vi "Trapu16toDbl.vi"(9 "Detector Type":string, 10 "Trap Sets":u32, 11 "Raw Trap Data In":i16[](array[numeric])) -> (0 "Channel pattern":i32, 1 "Channel Names":string[](array[string]), 2 "Trap Data":dbl[][](array[numeric]), 3 "Trap Data Out":i16[](array[numeric]))   [LabVIEW 2013]
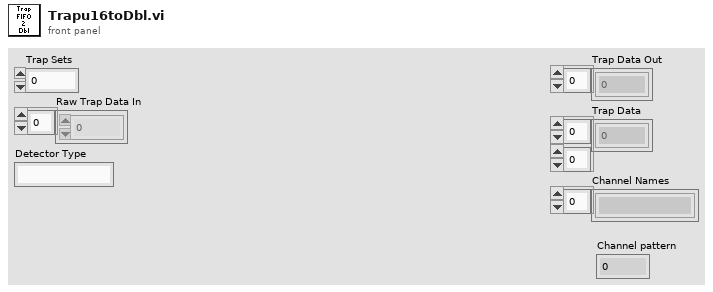
[diagram p1: front panel]
types:
  T1 = cluster{string, string, string, string, string, string, string, string}
  T2 = cluster{string, string, string, string, string, string, string, string, string, string, string, string}
  T3 = cluster{string, string, string, string, string, string, string, string, string, string, string, string, string}
  T4 = cluster{string, string, string, string, string, string, string, string, string, string, string, string, string, string}
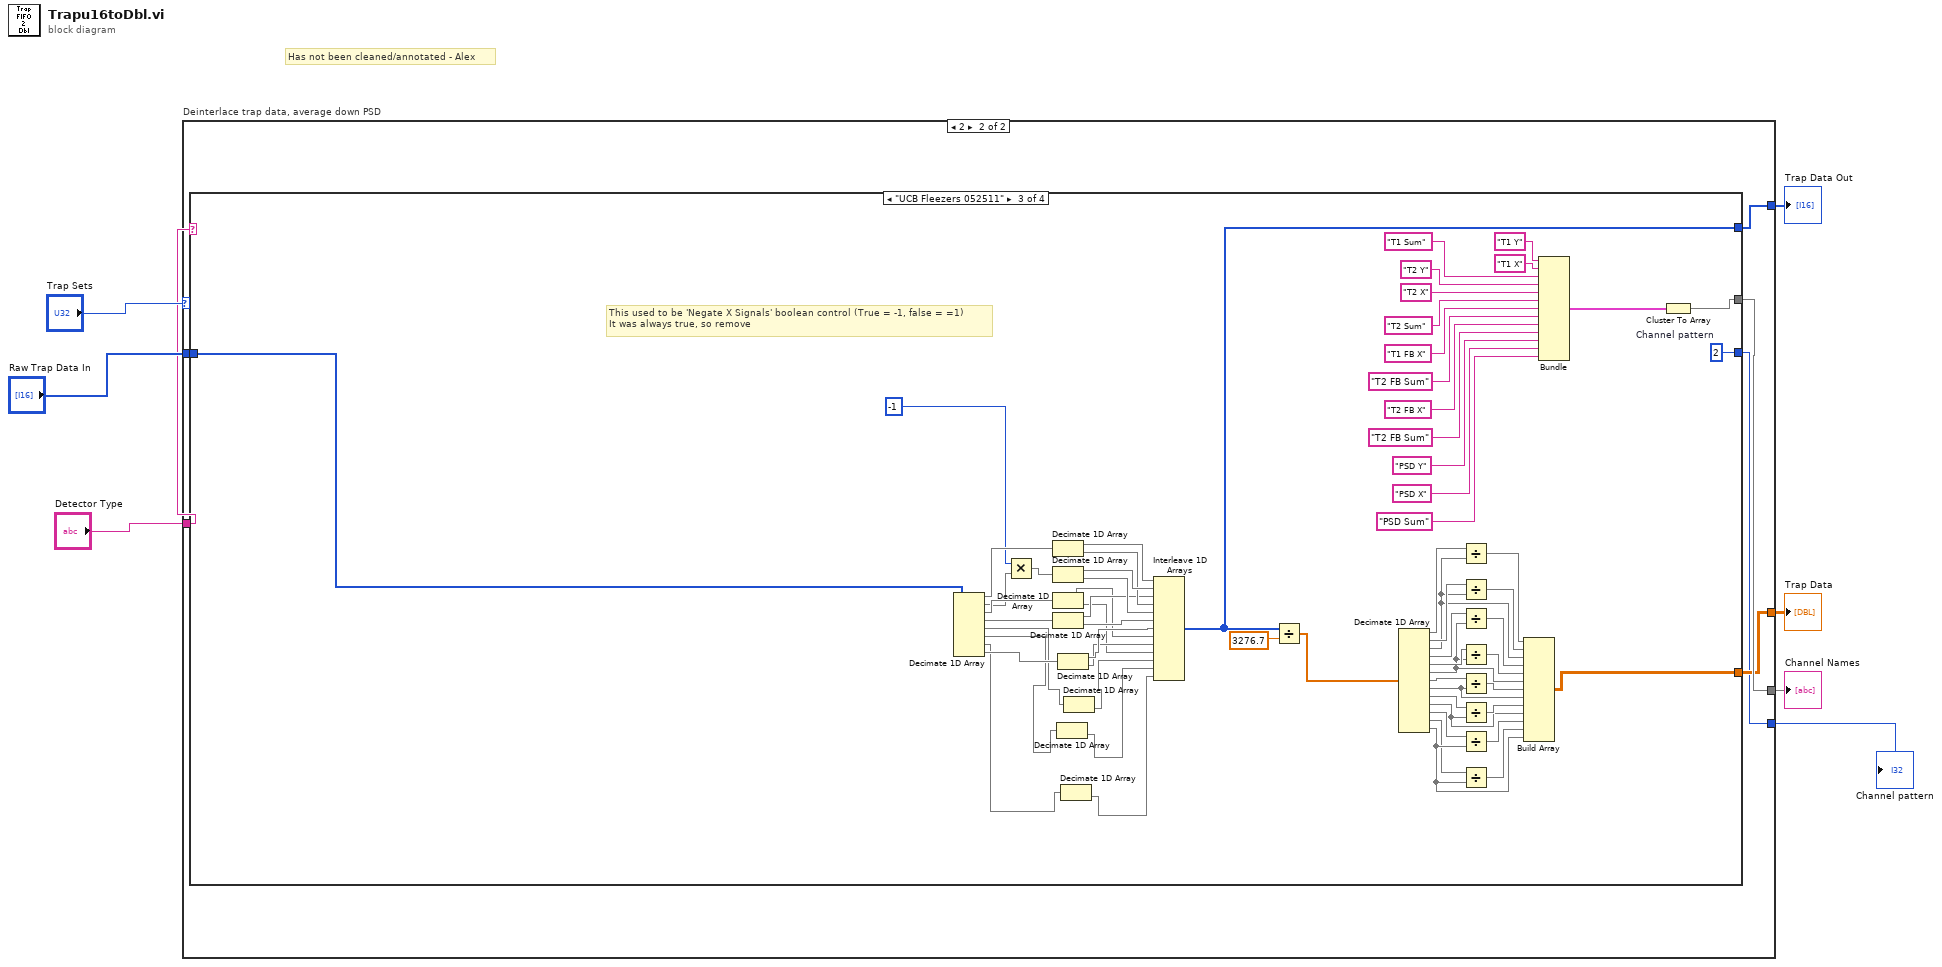
[diagram p0: block diagram]
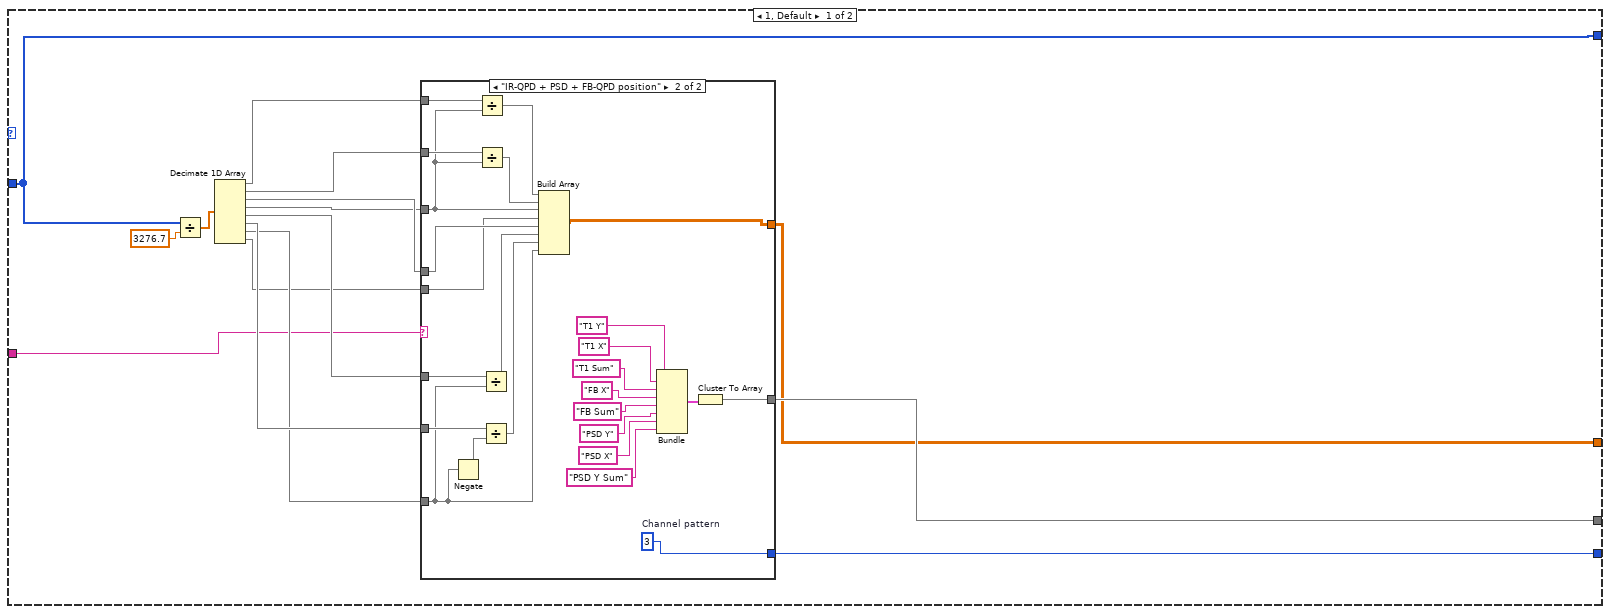
[diagram p2: hidden frame]
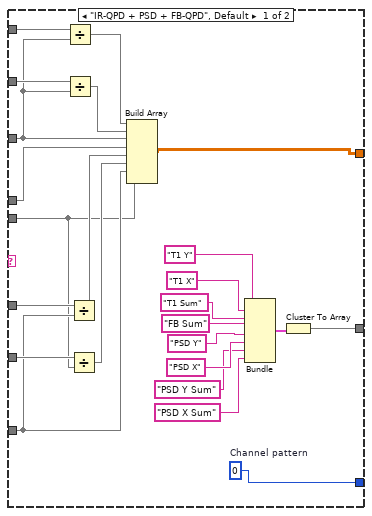
[diagram p3: hidden frame]
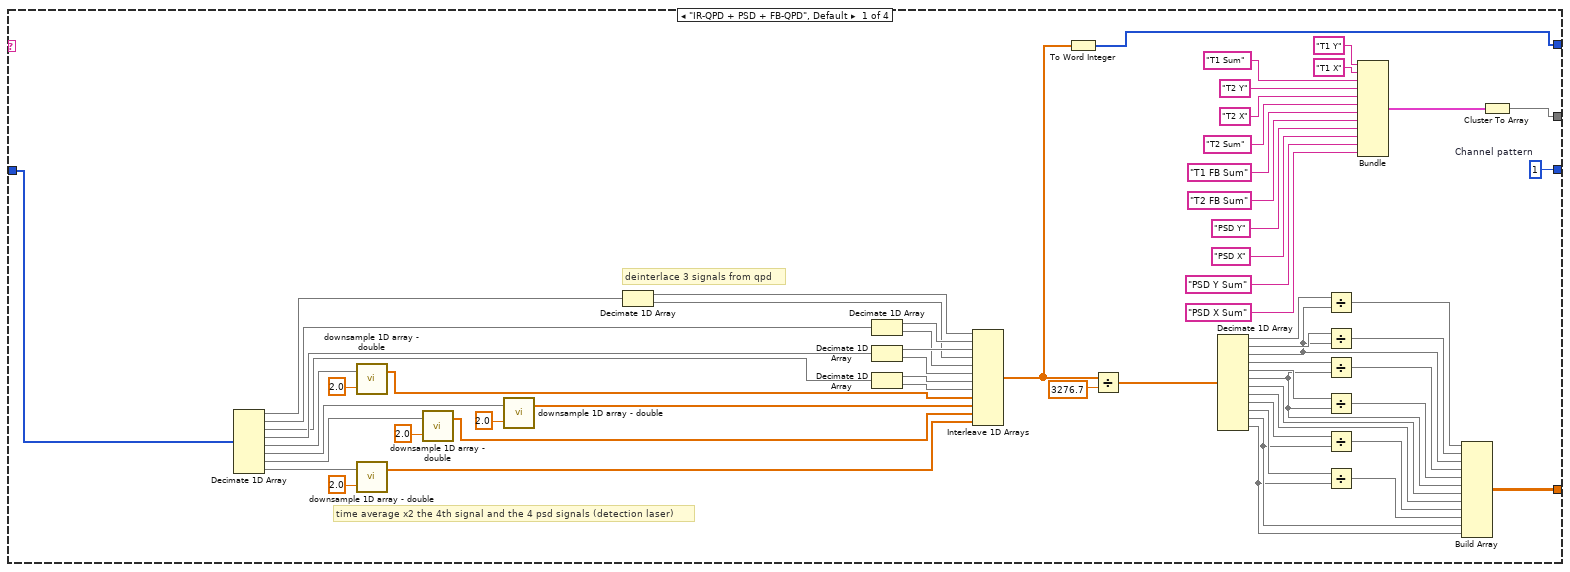
[diagram p4: hidden frame]
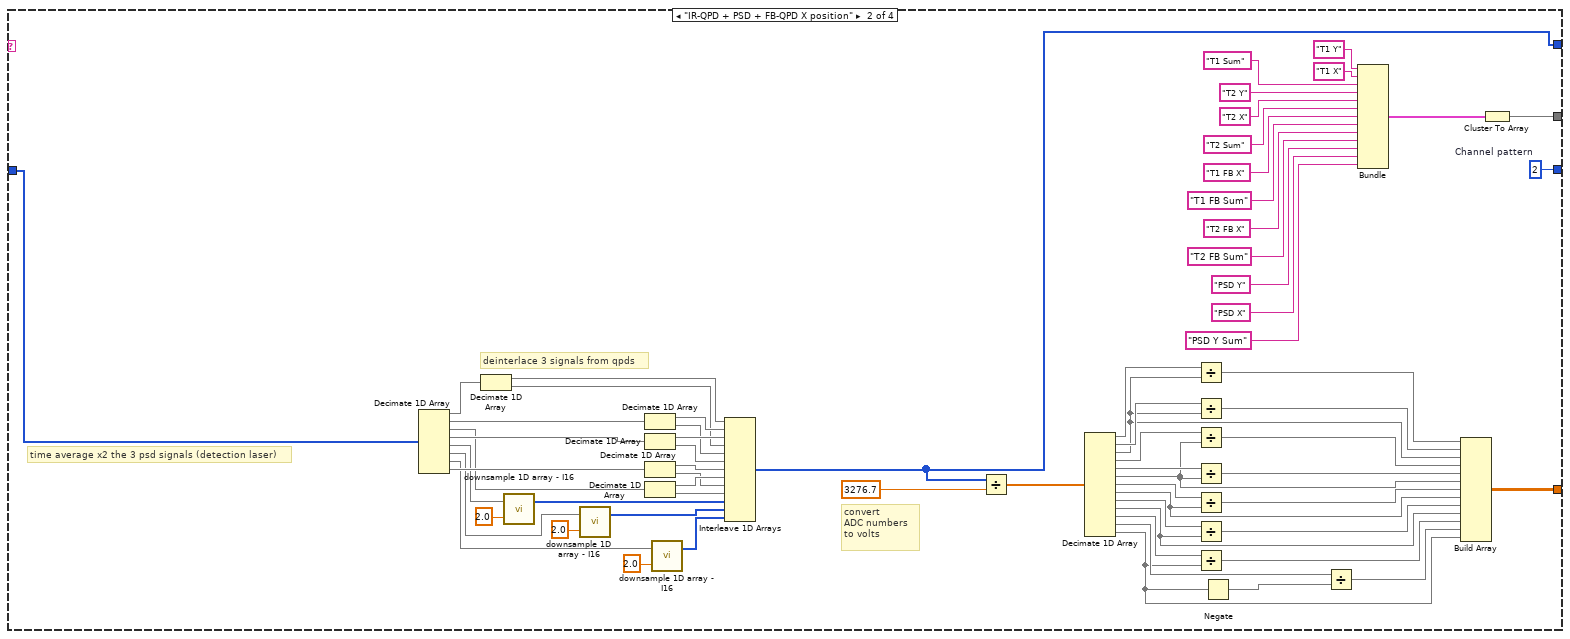
[diagram p5: hidden frame]
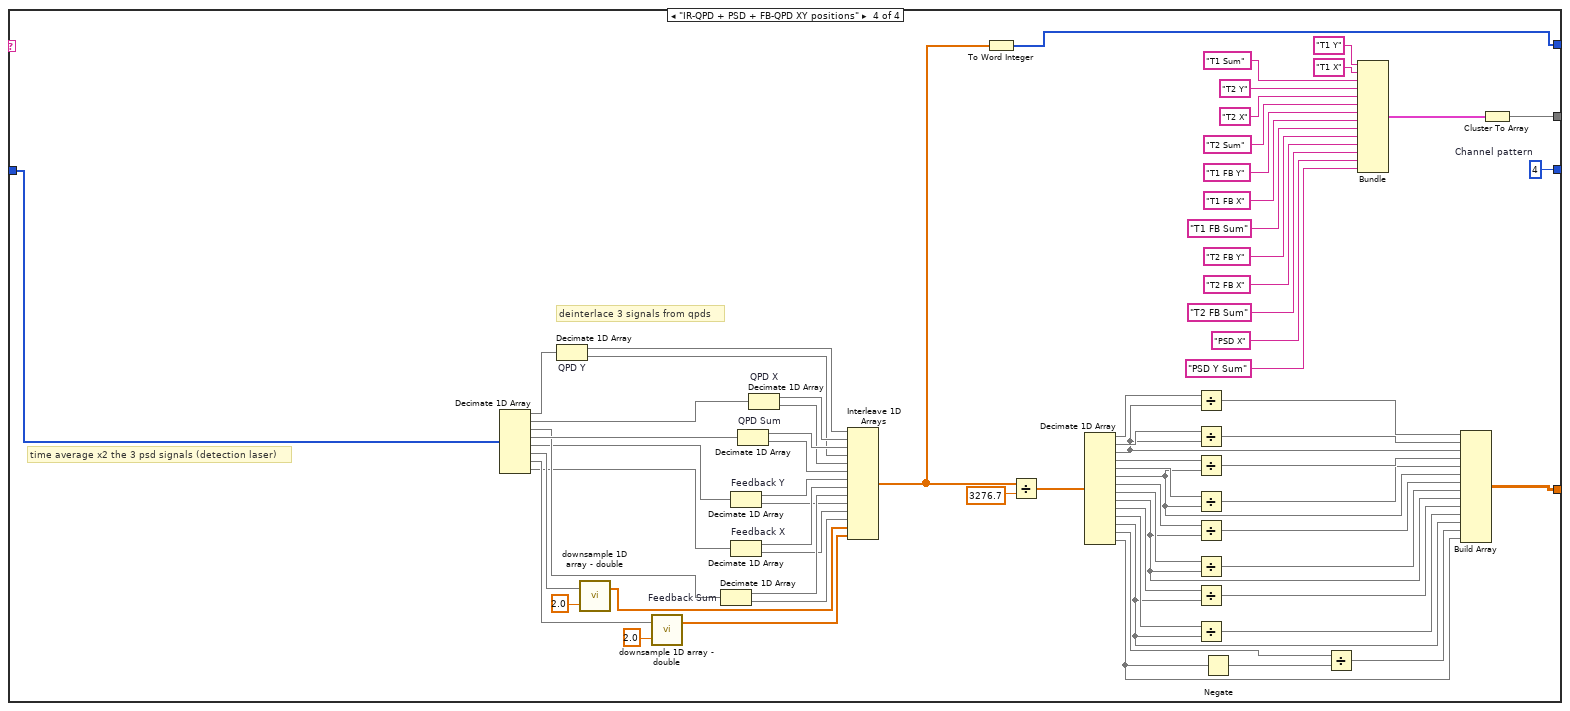
[diagram p6: hidden frame]
diagram:
  # "Has not been cleaned/annotated - Alex"
  n1 = case "Deinterlace trap data, average down PSD" shown="2" "Trap Sets" {
    tunnel: [w11 w75] -> w3
    tunnel: [w8 w77] -> w4
    tunnel: "Detector Type" -> [w13 w73]
    tunnel: [w12 w76] -> w2
    tunnel: [w10 w74] -> w1
    tunnel: "Raw Trap Data In" -> [w8 w72]
    frame 1, Default {
      n2 = Divide(x=w8, y=3276.7) -> (x/y=w9:dbl[])
      n3 = Decimate 1D Array(w9) -> (w22:dbl[], w21:dbl[], w20:dbl[], w19:dbl[], w18:dbl[], w17:dbl[], w16:dbl[], w15:dbl[])
      n4 = case shown="\"IR-QPD + PSD + FB-QPD position\"" w13 {
        tunnel: w22 -> [w46 w71]
        tunnel: w21 -> [w45 w70]
        tunnel: w20 -> [w30 w48]
        tunnel: w19 -> [w31 w58]
        tunnel: w18 -> [w44 w69]
        tunnel: w17 -> [w43 w68]
        tunnel: w16 -> [w27 w49]
        tunnel: w15 -> [w26 w47]
        tunnel: [w25 w55] -> w12
        tunnel: [w24 w54] -> w11
        tunnel: [w23 w53] -> w10
        frame "IR-QPD + PSD + FB-QPD", Default {
          w23 = 0  # Channel pattern
          n5 = Divide(x=w46, y=w31) -> (x/y=w33:dbl[])
          n6 = Divide(x=w45, y=w31) -> (x/y=w32:dbl[])
          n7 = Divide(x=w44, y=w27) -> (x/y=w29:dbl[])
          n8 = Divide(x=w43, y=w26) -> (x/y=w28:dbl[])
          n9 = Build Array(w33, w32, w31, w30, w29, w28, w27, w26) -> (w24:dbl[][])
          n10 = Bundle("T1 Y", "T1 X", "T1 Sum", "FB Sum", "PSD Y", "PSD X", "PSD Y Sum", "PSD X Sum") -> (w42:T1)  [unwired: 1 out]
          n11 = Cluster To Array(cluster=w42) -> (array=w25:string[])
        }
        frame "IR-QPD + PSD + FB-QPD position" {
          w53 = 3  # Channel pattern
          n12 = Negate(x=w49) -> (-x=w50:dbl[])
          n13 = Divide(x=w71, y=w58) -> (x/y=w60:dbl[])
          n14 = Divide(x=w70, y=w58) -> (x/y=w59:dbl[])
          n15 = Divide(x=w69, y=w49) -> (x/y=w57:dbl[])
          n16 = Divide(x=w68, y=w50) -> (x/y=w56:dbl[])
          n17 = Build Array(w60, w59, w58, w47, w48, w57, w56, w49) -> (w54:dbl[][])
          n18 = Bundle("T1 Y", "T1 X", "T1 Sum", "FB X", "FB Sum", "PSD Y", "PSD X", "PSD Y Sum") -> (w67:T1)  [unwired: 1 out]
          n19 = Cluster To Array(cluster=w67) -> (array=w55:string[])
        }
      }
    }
    frame 2 {
      n20 = case shown="\"UCB Fleezers 052511\"" w73 {
        tunnel: [w79 w199 w239 w274] -> w77
        tunnel: [w106 w190 w241 w321] -> w76
        tunnel: [w105 w154 w232 w288] -> w75
        tunnel: [w99 w189 w272 w319] -> w74
        tunnel: w72 -> [w78 w141 w209 w273]
        frame "IR-QPD + PSD + FB-QPD", Default {
          w99 = 1  # Channel pattern
          # "time average x2 the 4th signal and the 4 psd signals (detection laser)"
          # "deinterlace 3 signals from qpd"
          n21 = Decimate 1D Array(w78) -> (w139:i16[], w138:i16[], w104:i16[], w137:i16[], w127:i16[], w125:i16[], w124:i16[], w122:i16[])
          n22 = call "downsample 1D array - double.vi"("Ave N"=2.0, "Array In"=w127) -> ("Array Out"=w126:dbl[])  [unwired: 1 out]
          n23 = call "downsample 1D array - double.vi"("Ave N"=2.0, "Array In"=w122) -> ("Array Out"=w121:dbl[])  [unwired: 1 out]
          n24 = call "downsample 1D array - double.vi"("Ave N"=2.0, "Array In"=w124) -> ("Array Out"=w123:dbl[])  [unwired: 1 out]
          n25 = call "downsample 1D array - double.vi"("Ave N"=2.0, "Array In"=w125) -> ("Array Out"=w107:dbl[])  [unwired: 1 out]
          n26 = Decimate 1D Array(w139) -> (w136:i16[], w108:i16[])
          n27 = Decimate 1D Array(w138) -> (w135:i16[], w133:i16[])
          n28 = Decimate 1D Array(w137) -> (w134:i16[], w132:i16[])
          n29 = Decimate 1D Array(w104) -> (w103:i16[], w102:i16[])
          n30 = Interleave 1D Arrays(w136, w135, w134, w108, w133, w132, w103, w102, w126, w107, w123, w121) -> (w120:dbl[])
          n31 = To Word Integer(number=w120) -> (16bit integer=w79:i16[])
          n32 = Divide(x=w120, y=3276.7) -> (x/y=w119:dbl[])
          n33 = Decimate 1D Array(w119) -> (w118:dbl[], w117:dbl[], w116:dbl[], w115:dbl[], w114:dbl[], w113:dbl[], w101:dbl[], w100:dbl[], w112:dbl[], w111:dbl[], w110:dbl[], w109:dbl[])
          n34 = Divide(x=w118, y=w116) -> (x/y=w86:dbl[])
          n35 = Divide(x=w117, y=w116) -> (x/y=w85:dbl[])
          n36 = Divide(x=w115, y=w113) -> (x/y=w84:dbl[])
          n37 = Divide(x=w114, y=w113) -> (x/y=w83:dbl[])
          n38 = Divide(x=w112, y=w110) -> (x/y=w82:dbl[])
          n39 = Divide(x=w111, y=w109) -> (x/y=w81:dbl[])
          n40 = Bundle("T1 Y", "T1 X", "T1 Sum", "T2 Y", "T2 X", "T2 Sum", "T1 FB Sum", "T2 FB Sum", "PSD Y", "PSD X", "PSD Y Sum", "PSD X Sum") -> (w87:T2)  [unwired: 1 out]
          n41 = Build Array(w86, w85, w116, w84, w83, w113, w101, w100, w82, w81, w110, w109) -> (w105:dbl[][])
          n42 = Cluster To Array(cluster=w87) -> (array=w106:string[])
        }
        frame "IR-QPD + PSD + FB-QPD X position" {
          w189 = 2  # Channel pattern
          # "convert\nADC numbers\nto volts"
          # "time average x2 the 3 psd signals (detection laser)"
          # "deinterlace 3 signals from qpds"
          n43 = Decimate 1D Array(w141) -> (w206:i16[], w205:i16[], w142:i16[], w143:i16[], w152:i16[], w149:i16[], w146:i16[], w177:i16[])
          n44 = Decimate 1D Array(w206) -> (w204:i16[], w191:i16[])
          n45 = call "downsample 1D array - I16.vi"("Ave N"=2.0, "Array In"=w152) -> ("Array Out"=w150:i16[])  [unwired: 1 in]
          n46 = call "downsample 1D array - I16.vi"("Ave N"=2.0, "Array In"=w149) -> ("Array Out"=w147:i16[])  [unwired: 1 in]
          n47 = Decimate 1D Array(w205) -> (w203:i16[], w201:i16[])
          n48 = Decimate 1D Array(w143) -> (w202:i16[], w200:i16[])
          n49 = Decimate 1D Array(w177) -> (w176:i16[], w174:i16[])
          n50 = Decimate 1D Array(w142) -> (w175:i16[], w173:i16[])
          n51 = call "downsample 1D array - I16.vi"("Ave N"=2.0, "Array In"=w146) -> ("Array Out"=w144:i16[])  [unwired: 1 in]
          n52 = Interleave 1D Arrays(w204, w203, w202, w191, w201, w200, w176, w175, w174, w173, w150, w147, w144) -> (w199:i16[])
          n53 = Divide(x=w199, y=3276.7) -> (x/y=w198:dbl[])
          n54 = Decimate 1D Array(w198) -> (w197:dbl[], w196:dbl[], w195:dbl[], w194:dbl[], w193:dbl[], w192:dbl[], w165:dbl[], w163:dbl[], w162:dbl[], w160:dbl[], w159:dbl[], w158:dbl[], w155:dbl[])
          n55 = Divide(x=w197, y=w195) -> (x/y=w181:dbl[])
          n56 = Divide(x=w196, y=w195) -> (x/y=w180:dbl[])
          n57 = Divide(x=w194, y=w192) -> (x/y=w179:dbl[])
          n58 = Divide(x=w193, y=w192) -> (x/y=w178:dbl[])
          n59 = Divide(x=w165, y=w163) -> (x/y=w164:dbl[])
          n60 = Divide(x=w162, y=w160) -> (x/y=w161:dbl[])
          n61 = Divide(x=w159, y=w155) -> (x/y=w157:dbl[])
          n62 = Negate(x=w155) -> (-x=w153:dbl[])
          n63 = Divide(x=w158, y=w153) -> (x/y=w156:dbl[])
          n64 = Bundle("T1 Y", "T1 X", "T1 Sum", "T2 Y", "T2 X", "T2 Sum", "T1 FB X", "T1 FB Sum", "T2 FB X", "T2 FB Sum", "PSD Y", "PSD X", "PSD Y Sum") -> (w182:T3)  [unwired: 1 out]
          n65 = Build Array(w181, w180, w195, w179, w178, w192, w164, w163, w161, w160, w157, w156, w155) -> (w154:dbl[][])
          n66 = Cluster To Array(cluster=w182) -> (array=w190:string[])
        }
        frame "UCB Fleezers 052511" {
          w272 = 2  # Channel pattern
          # "This used to be 'Negate X Signals' boolean control (True = -1, false = =1)\nIt was always true, so remove"
          n67 = Decimate 1D Array(w209) -> (w217:i16[], w218:i16[], w226:i16[], w242:i16[], w215:i16[], w213:i16[], w211:i16[], w223:i16[])
          n68 = Multiply(x=i16 -1, y=w218) -> (x*y=w216:i16[])
          n69 = Decimate 1D Array(w217) -> (w270:i16[], w260:i16[])
          n70 = Decimate 1D Array(w216) -> (w269:i16[], w268:i16[])
          n71 = Decimate 1D Array(w226) -> (w220:i16[], w219:i16[])
          n72 = Decimate 1D Array(w242) -> (w225:i16[], w224:i16[])
          n73 = Decimate 1D Array(w213) -> (w212:i16[])  [unwired: 1 out]
          n74 = Decimate 1D Array(w223) -> (w222:i16[], w221:i16[])
          n75 = Decimate 1D Array(w211) -> (w210:i16[])  [unwired: 1 out]
          n76 = Decimate 1D Array(w215) -> (w214:i16[])  [unwired: 1 out]
          n77 = Interleave 1D Arrays(w270, w269, w225, w260, w268, w224, w222, w220, w221, w219, w214, w212, w210) -> (w239:i16[])
          n78 = Divide(x=w239, y=3276.7) -> (x/y=w267:dbl[])
          n79 = Decimate 1D Array(w267) -> (w266:dbl[], w265:dbl[], w264:dbl[], w263:dbl[], w262:dbl[], w261:dbl[], w238:dbl[], w236:dbl[], w235:dbl[], w233:dbl[], w231:dbl[], w228:dbl[], w229:dbl[])
          n80 = Divide(x=w266, y=w264) -> (x/y=w247:dbl[])
          n81 = Divide(x=w265, y=w264) -> (x/y=w246:dbl[])
          n82 = Divide(x=w263, y=w261) -> (x/y=w245:dbl[])
          n83 = Divide(x=w262, y=w261) -> (x/y=w244:dbl[])
          n84 = Divide(x=w238, y=w236) -> (x/y=w237:dbl[])
          n85 = Divide(x=w235, y=w233) -> (x/y=w234:dbl[])
          n86 = Divide(x=w231, y=w229) -> (x/y=w230:dbl[])
          n87 = Divide(x=w228, y=w229) -> (x/y=w227:dbl[])
          n88 = Build Array(w247, w246, w264, w245, w244, w261, w237, w236, w234, w233, w230, w227, w229) -> (w232:dbl[][])
          n89 = Bundle("T1 Y", "T1 X", "T1 Sum", "T2 Y", "T2 X", "T2 Sum", "T1 FB X", "T2 FB Sum", "T2 FB X", "T2 FB Sum", "PSD Y", "PSD X", "PSD Sum") -> (w248:T3)  [unwired: 1 out]
          n90 = Cluster To Array(cluster=w248) -> (array=w241:string[])
        }
        frame "IR-QPD + PSD + FB-QPD XY positions" {
          w319 = 4  # Channel pattern
          # "time average x2 the 3 psd signals (detection laser)"
          # "deinterlace 3 signals from qpds"
          n91 = Decimate 1D Array(w273) -> (w342:i16[], w341:i16[], w320:i16[], w340:i16[], w286:i16[], w332:i16[], w331:i16[], w308:i16[])
          n92 = Decimate 1D Array "QPD Y"(w342) -> (w339:i16[], w322:i16[])
          n93 = call "downsample 1D array - double.vi"("Ave N"=2.0, "Array In"=w332) -> ("Array Out"=w307:dbl[])  [unwired: 1 out]
          n94 = call "downsample 1D array - double.vi"("Ave N"=2.0, "Array In"=w331) -> ("Array Out"=w306:dbl[])  [unwired: 1 out]
          n95 = Decimate 1D Array "Feedback Sum"(w320) -> (w304:i16[], w302:i16[])
          n96 = Decimate 1D Array "Feedback Y"(w286) -> (w285:i16[], w284:i16[])
          n97 = Decimate 1D Array "Feedback X"(w308) -> (w305:i16[], w303:i16[])
          n98 = Decimate 1D Array "QPD Sum"(w340) -> (w337:i16[], w335:i16[])
          n99 = Decimate 1D Array "QPD X"(w341) -> (w338:i16[], w336:i16[])
          n100 = Interleave 1D Arrays(w339, w338, w337, w322, w336, w335, w285, w305, w304, w284, w303, w302, w307, w306) -> (w330:dbl[])
          n101 = To Word Integer(number=w330) -> (16bit integer=w274:i16[])
          n102 = Divide(x=w330, y=3276.7) -> (x/y=w329:dbl[])
          n103 = Decimate 1D Array(w329) -> (w328:dbl[], w327:dbl[], w326:dbl[], w325:dbl[], w324:dbl[], w323:dbl[], w281:dbl[], w295:dbl[], w279:dbl[], w280:dbl[], w293:dbl[], w277:dbl[], w291:dbl[], w289:dbl[])
          n104 = Divide(x=w328, y=w326) -> (x/y=w312:dbl[])
          n105 = Divide(x=w327, y=w326) -> (x/y=w311:dbl[])
          n106 = Divide(x=w325, y=w323) -> (x/y=w310:dbl[])
          n107 = Divide(x=w324, y=w323) -> (x/y=w309:dbl[])
          n108 = Divide(x=w281, y=w279) -> (x/y=w278:dbl[])
          n109 = Divide(x=w295, y=w279) -> (x/y=w294:dbl[])
          n110 = Divide(x=w280, y=w277) -> (x/y=w276:dbl[])
          n111 = Divide(x=w293, y=w277) -> (x/y=w292:dbl[])
          n112 = Negate(x=w289) -> (-x=w287:dbl[])
          n113 = Divide(x=w291, y=w287) -> (x/y=w290:dbl[])
          n114 = Bundle("T1 Y", "T1 X", "T1 Sum", "T2 Y", "T2 X", "T2 Sum", "T1 FB Y", "T1 FB X", "T1 FB Sum", "T2 FB Y", "T2 FB X", "T2 FB Sum", "PSD X", "PSD Y Sum") -> (w275:T4)  [unwired: 1 out]
          n115 = Build Array(w312, w311, w326, w310, w309, w323, w278, w294, w279, w276, w292, w277, w290, w289) -> (w288:dbl[][])
          n116 = Cluster To Array(cluster=w275) -> (array=w321:string[])
        }
      }
    }
  }
  "Trap Data Out" <- w4
  "Trap Data" <- w3
  "Channel Names" <- w2
  "Channel pattern" <- w1
